vi "Analog_Yaw.vi"(11 "Gyro":T1) -> (3 "Analog_Yaw":dbl)   [LabVIEW 2014]
uses:
  <vilib>/Rock Robotics/WPI/Gyro/WPI_GyroDevRef.ctl
  <vilib>/Rock Robotics/SystemInterfaces/Typedef/FPGA_TypedefAnalogModule.ctl
  <vilib>/Rock Robotics/SystemInterfaces/AI/FPGA_AIChannel.ctl
panel:
  in  "Reset Zero Position in":bool
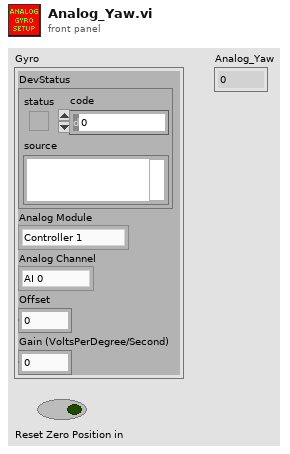
[diagram p1: front panel]
types:
  T1 = typedef "WPI_GyroDevRef.ctl" = cluster{"DevStatus":errorcluster, "Analog Module":T2, "Analog Channel":T3, "Offset":dbl, "Gain (VoltsPerDegree/Second)":dbl}
  T2 = typedef "FPGA_TypedefAnalogModule.ctl" = enum16{"Controller 1"}
  T3 = typedef "FPGA_AIChannel.ctl" = enum8{"AI 0", "AI 1", "AI 2", "AI 3", "AI MXP 0", "AI MXP 1", "AI MXP 2", "AI MXP 3", "Invalid"}
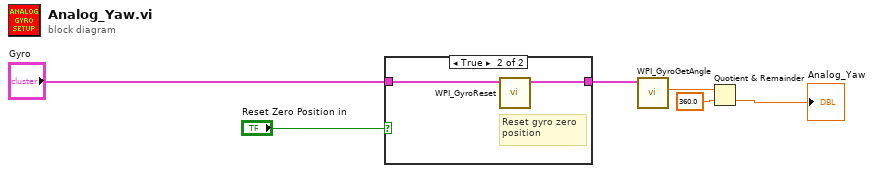
[diagram p0: block diagram]
diagram:
  n1 = case shown="True" "Reset Zero Position in" {
    tunnel: [w7 w9] -> w5
    tunnel: "Gyro" -> [w7 w8]
    frame False {
    }
    frame True {
      # "Reset gyro zero \nposition"
      n2 = call <vilib>:"WPI_GyroReset.vi"("GyroDevRef"=w8) -> ("GyroDevRef"=w9:T1)  [unwired: 10 out]
    }
  }
  n3 = call <vilib>:"WPI_GyroGetAngle.vi"("GyroDevRef"=w5) -> ("Angle"=w4:dbl)  [unwired: 1 in, 9 out]
  n4 = Quotient & Remainder(x=w4, y=360.0) -> (floor(x/y)=→"Analog_Yaw":dbl)  [unwired: 1 out]
